vi "compound_arithmatic.vi"() -> ()   [LabVIEW 2019]
panel:
  out "result":dbl
  in  "Numeric 5":dbl
  in  "Numeric 4":dbl
  in  "Numeric 3":dbl
  in  "Numeric 2":dbl
  in  "Numeric":dbl
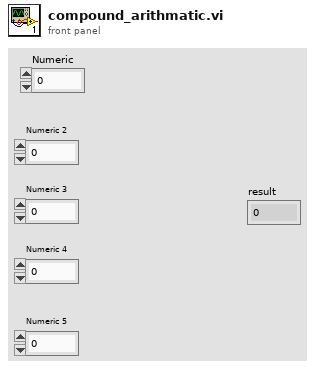
[diagram p1: front panel]
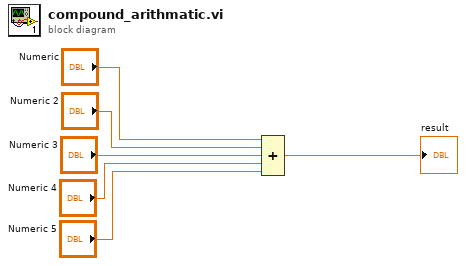
[diagram p0: block diagram]
diagram:
  n1 = Compound Arithmetic op=ADD("Numeric", "Numeric 2", "Numeric 3", "Numeric 4", "Numeric 5") -> (→"result":dbl)
